vi "RX JESD Sync.vi"(0 "rx baseband session in":T2={"3630 session"={"VISA resource name"="", "Address Space"=1, "window_offset"=0, "register_addresses"={"MM based Registers"={"Revision"=0, "OldestCompatRev"=0, "signature"=0, "scratch"=0, "LedControl"=0, "BoardHwRev"=0, "BoardControl"=0, "ThermalStatus"=0, "BasebandStatus"=0, "BasebandControl"=0, "BasebandAuxSetup"=0, "BasebandAuxStatus"=0, "LmkSyncOutSetup"=0, " AdcSyncOutSetup"=0, " InjSyncOutSetup"=0, " PxiTrig0OutSetup"=0, " PxiTrig1OutSetup"=0, " PxiTrig2OutSetup"=0, " PxiTrig3OutSetup"=0, " PxiTrig4OutSetup"=0, " PxiTrig5OutSetup"=0, " PxiTrig6OutSetup"=0, " PxiTrig7OutSetup"=0}, "CPLD based Registers"={"SlaveSignature"=0, "SlaveRevision"=0, "SlaveOldestCompatRev"=0, "SlaveScratch"=0, "SlaveSetup"=0, "SlaveStatus"=0, "IDacReg_offset"=0, "LMKRegGrp0_offset"=0, "QDacReg_offset"=0, "BrdTempSensorVal"=0, "TempSensorPowerDown"=0, "GPIOReg_offset"=0, "IAdcReg_offset"=0, "QAdcReg_offset"=0, "LMKRegGrp1_offset"=0, "QadcTempSensorVal"=0, "IadcTempSensorVal"=0, "RevisionReg"=0, "VcxoReg"=0, "CpldStatusReg"=0, "PowerReg"=0, "VBiasEnReg"=0, "ExtRefOeReg"=0, "QdacCtrlReg"=0, "QdacStatusReg"=0, "IdacCtrlReg"=0, "IdacStatusReg"=0, "QdacJtagIn"=0, "QdacJtagOut"=0, "IdacJtagIn"=0, "IdacJtagOut"=0, "IqDcSetupReg"=0, "QadcStatusReg"=0, "IadcStatusReg"=0, "BrdSetupReg"=0, "IqDcRevisionReg"=0, "PllStatusReg"=0, "EndpointScratchReg"=0, "AdcSyncCfgReg"=0, "IqCardOpampReg"=0}, "CPLD Register Offset"=0, "MM  Register Offset"=0, " PxiTrig0OutSetup"=0}, "required_MM_fpga_version"={"signature"=0, "hardware"=0, "current revision"=0, "oldest revision"=0}, "CPLD Oldest Compat Version "={"hardware"=0, "CPLD firmware"=0}, "MM_FPGA_image_location"="", "is_init"=FALSE, "card_type"=enum."ADC", "DacLmkConfigFileName"="", "AdcLmkConfigFileName"="", "AdcConfigFileName"="", "DacConfigFileName_RevA"="", "DacConfigFileName_RevB"="", "Mulde hardware revision"=0, "bypass DAC PLL\n"=FALSE, "IQ Card Revision"=enum."RevA", "board capability"={"baseband sync"=enum."no baseband sync"}}, "7902 reference"=refnum} {"3630 session"."Address Space" items=["VXI/VME A16"=1, "VXI/VME A24"=2, "VXI/VME A32"=3, "VXI/VME A64"=4, "PXI Memory Allocations"=9, "PXI Configuration"=10, "PXI BAR0"=11, "PXI BAR1"=12, "PXI BAR2"=13, "PXI BAR3"=14, "PXI BAR4"=15, "PXI BAR5"=16]}, 5 "fpga reference in":refnum<k20>[](array[refnum]), 7 "direction":T1, 9 "timeout (ms)":dbl=500.0 format="%#_13g", 11 "error in":errorcluster) -> (4 "rx baseband session out":T2={"3630 session"={"VISA resource name"="", "Address Space"=1, "window_offset"=0, "register_addresses"={"MM based Registers"={"Revision"=0, "OldestCompatRev"=0, "signature"=0, "scratch"=0, "LedControl"=0, "BoardHwRev"=0, "BoardControl"=0, "ThermalStatus"=0, "BasebandStatus"=0, "BasebandControl"=0, "BasebandAuxSetup"=0, "BasebandAuxStatus"=0, "LmkSyncOutSetup"=0, " AdcSyncOutSetup"=0, " InjSyncOutSetup"=0, " PxiTrig0OutSetup"=0, " PxiTrig1OutSetup"=0, " PxiTrig2OutSetup"=0, " PxiTrig3OutSetup"=0, " PxiTrig4OutSetup"=0, " PxiTrig5OutSetup"=0, " PxiTrig6OutSetup"=0, " PxiTrig7OutSetup"=0}, "CPLD based Registers"={"SlaveSignature"=0, "SlaveRevision"=0, "SlaveOldestCompatRev"=0, "SlaveScratch"=0, "SlaveSetup"=0, "SlaveStatus"=0, "IDacReg_offset"=0, "LMKRegGrp0_offset"=0, "QDacReg_offset"=0, "BrdTempSensorVal"=0, "TempSensorPowerDown"=0, "GPIOReg_offset"=0, "IAdcReg_offset"=0, "QAdcReg_offset"=0, "LMKRegGrp1_offset"=0, "QadcTempSensorVal"=0, "IadcTempSensorVal"=0, "RevisionReg"=0, "VcxoReg"=0, "CpldStatusReg"=0, "PowerReg"=0, "VBiasEnReg"=0, "ExtRefOeReg"=0, "QdacCtrlReg"=0, "QdacStatusReg"=0, "IdacCtrlReg"=0, "IdacStatusReg"=0, "QdacJtagIn"=0, "QdacJtagOut"=0, "IdacJtagIn"=0, "IdacJtagOut"=0, "IqDcSetupReg"=0, "QadcStatusReg"=0, "IadcStatusReg"=0, "BrdSetupReg"=0, "IqDcRevisionReg"=0, "PllStatusReg"=0, "EndpointScratchReg"=0, "AdcSyncCfgReg"=0, "IqCardOpampReg"=0}, "CPLD Register Offset"=0, "MM  Register Offset"=0, " PxiTrig0OutSetup"=0}, "required_MM_fpga_version"={"signature"=0, "hardware"=0, "current revision"=0, "oldest revision"=0}, "CPLD Oldest Compat Version "={"hardware"=0, "CPLD firmware"=0}, "MM_FPGA_image_location"="", "is_init"=FALSE, "card_type"=enum."ADC", "DacLmkConfigFileName"="", "AdcLmkConfigFileName"="", "AdcConfigFileName"="", "DacConfigFileName_RevA"="", "DacConfigFileName_RevB"="", "Mulde hardware revision"=0, "bypass DAC PLL\n"=FALSE, "IQ Card Revision"=enum."RevA", "board capability"={"baseband sync"=enum."no baseband sync"}}, "7902 reference"=refnum} {"3630 session"."Address Space" items=["VXI/VME A16"=1, "VXI/VME A24"=2, "VXI/VME A32"=3, "VXI/VME A64"=4, "PXI Memory Allocations"=9, "PXI Configuration"=10, "PXI BAR0"=11, "PXI BAR1"=12, "PXI BAR2"=13, "PXI BAR3"=14, "PXI BAR4"=15, "PXI BAR5"=16]}, 8 "timeout error":bool, 15 "error out":errorcluster)   [LabVIEW 2019]
uses:
  TypeDefs/Rx Baseband Session.ctl
  <instrlib>/niMmWave/ni3610 and ni3630/controls/public/Main Settings.ctl
  <vilib>/Instr/_visa.llb/VISA Register Access Address Space.ctl
  <instrlib>/niMmWave/ni3610 and ni3630/controls/public/Register Adresses.ctl
  <instrlib>/niMmWave/ni3610 and ni3630/controls/public/Base Card Type.ctl
  <instrlib>/niMmWave/ni3610 and ni3630/controls/private/IQ Card Revision.ctl
  <instrlib>/niMmWave/ni3610 and ni3630/controls/public/Board Capability.ctl
  TypeDefs/Blank FPGA Reference.ctl
  TypeDefs/Direction.ctl
  TypeDefs/RX FPGA Reference.ctl
  <vilib>/rvi/errors/niLvFpgaAdjustHostInterfaceError.vi
  <vilib>/rvi/interface/nirviReadWriteControl/nirviReadWriteControl.xnode
  <vilib>/rvi/interface/Simulation/niFpgaSimulationCallBeginRW.vi
  <instrlib>/niMmWave/ni3610 and ni3630/ni3610_and_ni3630_Driver_Lib.lvlib
  NiFpgaLv.dll
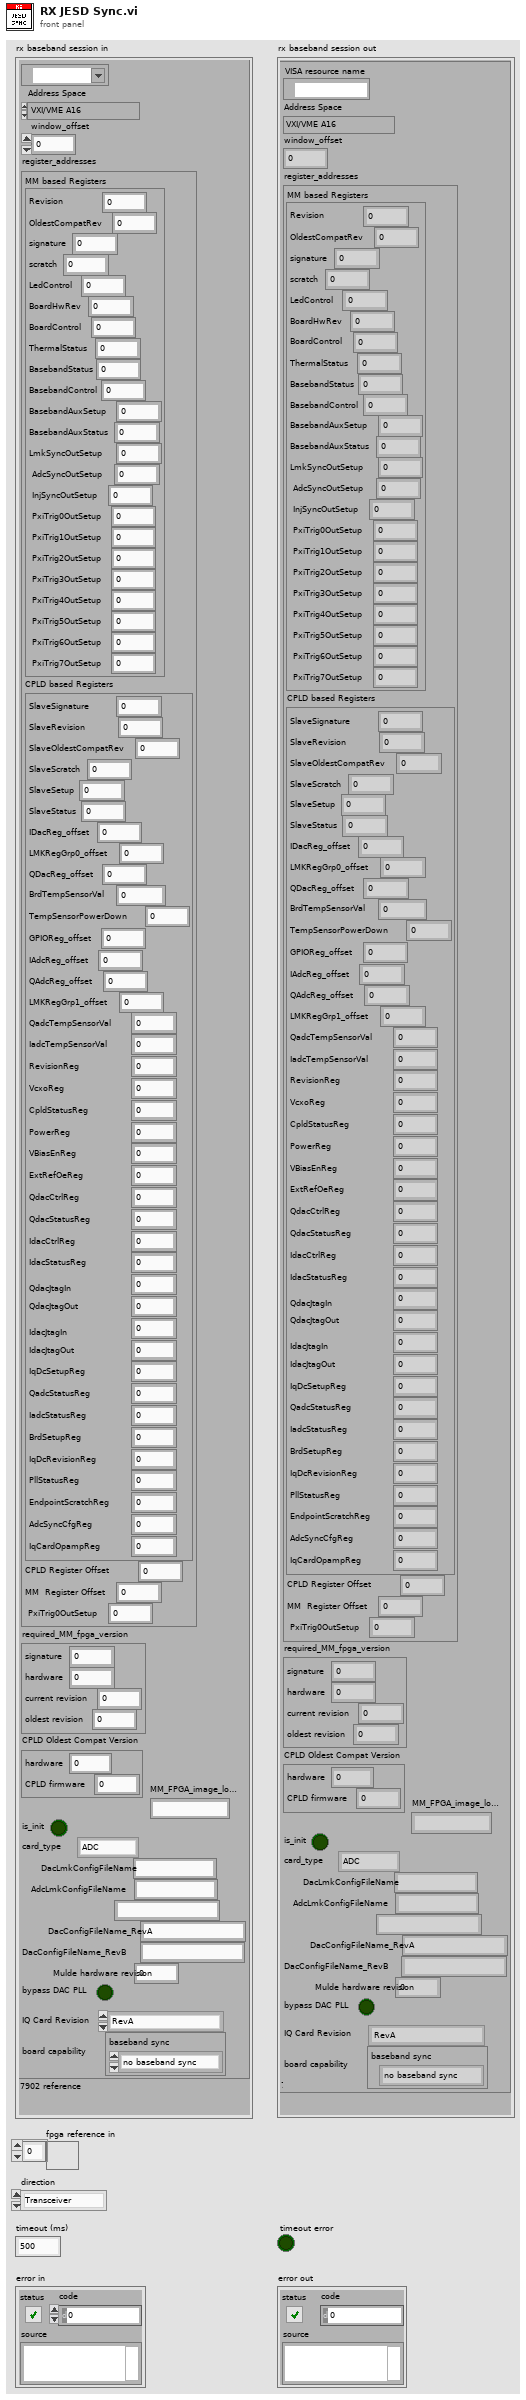
[diagram p1: front panel]
types:
  T1 = typedef "Direction.ctl" = enum16{"Transceiver", "Receiver", "Transmitter"}
  T2 = typedef "Rx Baseband Session.ctl" = cluster{"3630 session":T3, "7902 reference":T9}
  T3 = typedef "ni3610_and_ni3630_Driver_Lib.lvlib/Main Settings.ctl" = cluster{"VISA resource name":refnum<visa-resource-name>, "Address Space":T4, "window_offset":u32, "register_addresses":T5, "required_MM_fpga_version":cluster{"signature":u32, "hardware":u32, "current revision":u32, "oldest revision":u32}, "CPLD Oldest Compat Version ":cluster{"hardware":u32, "CPLD firmware":u32}, "MM_FPGA_image_location":string, "is_init":bool, "card_type":T6, "DacLmkConfigFileName":string, "AdcLmkConfigFileName":string, "AdcConfigFileName":string, "DacConfigFileName_RevA":string, "DacConfigFileName_RevB":string, "Mulde hardware revision":u8, "bypass DAC PLL\n":bool, "IQ Card Revision":T7, "board capability":T8}
  T4 = typedef "VISA Register Access Address Space.ctl" = u16
  T5 = typedef "ni3610_and_ni3630_Driver_Lib.lvlib/Register Adresses.ctl" = cluster{"MM based Registers":cluster{"Revision":u32, "OldestCompatRev":u32, "signature":u32, "scratch":u32, "LedControl":u32, "BoardHwRev":u32, "BoardControl":u32, "ThermalStatus":u32, "BasebandStatus":u32, "BasebandControl":u32, "BasebandAuxSetup":u32, "BasebandAuxStatus":u32, "LmkSyncOutSetup":u32, " AdcSyncOutSetup":u32, " InjSyncOutSetup":u32, " PxiTrig0OutSetup":u32, " PxiTrig1OutSetup":u32, " PxiTrig2OutSetup":u32, " PxiTrig3OutSetup":u32, " PxiTrig4OutSetup":u32, " PxiTrig5OutSetup":u32, " PxiTrig6OutSetup":u32, " PxiTrig7OutSetup":u32}, "CPLD based Registers":cluster{"SlaveSignature":u32, "SlaveRevision":u32, "SlaveOldestCompatRev":u32, "SlaveScratch":u32, "SlaveSetup":u32, "SlaveStatus":u32, "IDacReg_offset":u32, "LMKRegGrp0_offset":u32, "QDacReg_offset":u32, "BrdTempSensorVal":u32, "TempSensorPowerDown":u32, "GPIOReg_offset":u32, "IAdcReg_offset":u32, "QAdcReg_offset":u32, "LMKRegGrp1_offset":u32, "QadcTempSensorVal":u32, "IadcTempSensorVal":u32, "RevisionReg":u32, "VcxoReg":u32, "CpldStatusReg":u32, "PowerReg":u32, "VBiasEnReg":u32, "ExtRefOeReg":u32, "QdacCtrlReg":u32, "QdacStatusReg":u32, "IdacCtrlReg":u32, "IdacStatusReg":u32, "QdacJtagIn":u32, "QdacJtagOut":u32, "IdacJtagIn":u32, "IdacJtagOut":u32, "IqDcSetupReg":u32, "QadcStatusReg":u32, "IadcStatusReg":u32, "BrdSetupReg":u32, "IqDcRevisionReg":u32, "PllStatusReg":u32, "EndpointScratchReg":u32, "AdcSyncCfgReg":u32, "IqCardOpampReg":u32}, "CPLD Register Offset":u32, "MM  Register Offset":u32, " PxiTrig0OutSetup":u32}
  T6 = typedef "ni3610_and_ni3630_Driver_Lib.lvlib/Base Card Type.ctl" = enum16{"unspecified", "ADC", "DAC"}
  T7 = typedef "ni3610_and_ni3630_Driver_Lib.lvlib/IQ Card Revision.ctl" = enum16{"RevA", "RevB", "RevC", "RevD"}
  T8 = typedef "ni3610_and_ni3630_Driver_Lib.lvlib/Board Capability.ctl" = cluster{"baseband sync":enum16{"no baseband sync", "baseband sync"}}
  T9 = typedef "Blank FPGA Reference.ctl" = refnum<k20>
  T10 = typedef "RX FPGA Reference.ctl" = refnum<k20>
  T11 = cluster{"gtx enable":bool, "jesd enable":bool, "sw sync":bool, "buffer enable":bool, "clock enable":bool, "trig5 output enable":bool, "trig5 invert":bool}
  T12 = cluster{"gtx active":bool, "jesd active":bool, "lane sync req":bool, "lanes synced":bool, "lanes aligned":bool, "qpll locked":bool, "qpll ref lost":bool, "k-char error":bool, "lane alignment error":bool, "8b10b error":bool, "8b10b disparity error":bool, "buffer overflow":bool, "buffer underflow":bool, "buffer ready":bool, "mgt ref clocks locked":bool, "mgt ref clock valid":bool, "config complete":bool}
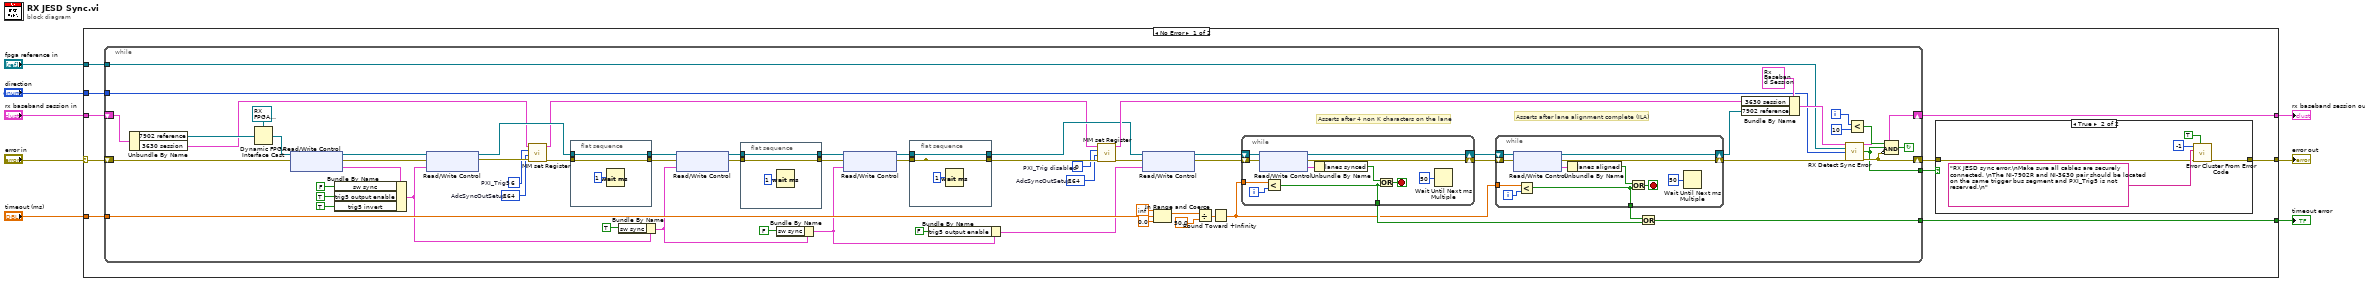
[diagram p0: block diagram]
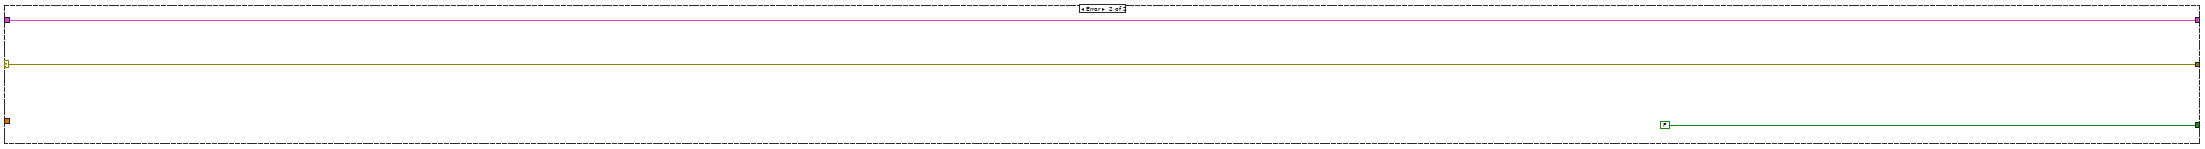
[diagram p3: hidden frame]
diagram:
  n1 = case shown="No Error" "error in" {
    selector: "error in" -> [w15 w124]
    tunnel: [w12 w124] -> w8
    tunnel: [w18 FALSE] -> w6
    tunnel: "timeout (ms)" -> [w17 _]
    tunnel: "rx baseband session in" -> [w16 w122]
    tunnel: [w11 w122] -> w3
    tunnel: "fpga reference in" -> [w10 _]
    tunnel: "direction" -> [w9 _]
    frame No Error {
      n2 = while {
        tunnel: [w80] -> w18
        tunnel: w17 -> [w79]
        shift-right: [w66] -> w13
        shift-left: w15 -> [w22]
        shift-right: [w56] -> w11
        shift-left: w16 -> [w58]
        tunnel: [w64] -> w14
        tunnel: w10 -> [w20]
        tunnel: w9 -> [w19]
        i -> [w65]
        stop <- w67 continue-if-true
        w38 = u32 0  # PXI_Trig disabled
        w37 = u32 264  # AdcSyncOutSetup
        w43 = u32 6  # PXI_Trig5
        w42 = u32 264  # AdcSyncOutSetup
        # "Asserts after lane alignment complete (ILA)"
        # "Asserts after 4 non K characters on the lane"
        n3 = Unbundle By Name(w58) -> ("7902 reference"=w60:T9, "3630 session"=w21:T3)
        n4 = Dynamic FPGA Interface Cast(Session In=T10 refnum ("fpga reference"), Type=w60) -> (Session Out=w36:T10)
        n5 = xnode "Read/Write Control"("FPGA VI Reference In"=w36, "error in"=w22) -> ("FPGA VI Reference Out"=w35:T10, "error out"=w34:errorcluster, "rxjesd.control"=w33:T11)
        n6 = Bundle By Name(cluster=w33, "sw sync"=FALSE ("txjesd.reset"), "trig5 output enable"=TRUE ("pxi trig 5 output enable"), "trig5 invert"=TRUE ("invert jesd sync to pin")) -> (w29:T11)
        n7 = xnode "Read/Write Control"("FPGA VI Reference In"=w35, "error in"=w34, "rxjesd.control"=w29) -> ("FPGA VI Reference Out"=w55:T10, "error out"=w44:errorcluster)
        n8 = call <instrlib>:"MM set Register.vi"("error in"=w44, "MM address"=w42, "Value"=w43, "Board Settings in"=w21) -> ("error out"=w45:errorcluster, "Board Settings out"=w39:T3)  [unwired: 6 in]
        n9 = flat-sequence {
          tunnel: w55 -> [w89]
          tunnel: w45 -> [w88]
          tunnel: [w89] -> w48
          tunnel: [w88] -> w49
          frame #0 {
            n10 = Wait (ms)(milliseconds to wait=u32 1) -> ()  [unwired: 1 out]
          }
        }
        n11 = Bundle By Name(cluster=w29, "sw sync"=TRUE ("rxjesd.sw sync")) -> (w25:T11)
        n12 = xnode "Read/Write Control"("FPGA VI Reference In"=w48, "error in"=w49, "rxjesd.control"=w25) -> ("FPGA VI Reference Out"=w52:T10, "error out"=w53:errorcluster)
        n13 = flat-sequence {
          tunnel: w52 -> [w92]
          tunnel: w53 -> [w91]
          tunnel: [w92] -> w51
          tunnel: [w91] -> w50
          frame #0 {
            n14 = Wait (ms)(milliseconds to wait=u32 1) -> ()  [unwired: 1 out]
          }
        }
        n15 = Bundle By Name(cluster=w25, "sw sync"=FALSE ("rxjesd.sw sync")) -> (w23:T11)
        n16 = xnode "Read/Write Control"("FPGA VI Reference In"=w51, "error in"=w50, "rxjesd.control"=w23) -> ("FPGA VI Reference Out"=w46:T10, "error out"=w47:errorcluster)
        n17 = flat-sequence {
          tunnel: w46 -> [w86]
          tunnel: [w85] -> _
          tunnel: [w86] -> w54
          tunnel: [w85] -> w40
          tunnel: w47 -> [w85]
          frame #0 {
            n18 = Wait (ms)(milliseconds to wait=u32 1) -> ()  [unwired: 1 out]
          }
        }
        n19 = Bundle By Name(cluster=w23, "trig5 output enable"=FALSE ("rxjesd.sw sync")) -> (w24:T11)
        n20 = call <instrlib>:"MM set Register.vi"("error in"=w40, "MM address"=w37, "Value"=w38, "Board Settings in"=w39) -> ("error out"=w41:errorcluster, "Board Settings out"=w63:T3)  [unwired: 6 in]
        n21 = xnode "Read/Write Control"("FPGA VI Reference In"=w54, "error in"=w41, "rxjesd.control"=w24) -> ("FPGA VI Reference Out"=w72:T10, "error out"=w71:errorcluster)
        n22 = In Range and Coerce(upper limit=inf, x=w79, lower limit=0.0) -> (coerced(x)=w76:dbl)  [unwired: 1 out]
        n23 = Divide(x=w76, y=50.0) -> (x/y=w74:dbl)
        n24 = Round Toward +Infinity(x=w74) -> (ceil(x): smallest int >= x=w73:dbl)
        n25 = while {
          shift-right: [w100] -> w83
          shift-left: w71 -> [w102]
          shift-right: [w103] -> w84
          shift-left: w72 -> [w104]
          tunnel: w73 -> [w97]
          tunnel: [w96] -> w82
          i -> [w99]
          stop <- w98 stop-if-true
          n26 = xnode "Read/Write Control"("FPGA VI Reference In"=w104, "error in"=w102) -> ("FPGA VI Reference Out"=w103:T10, "error out"=w100:errorcluster, "rxjesd.status"=w95:T12)
          n27 = Less?(x=w97, y=w99) -> (x < y?=w96:bool)
          n28 = Unbundle By Name(w95) -> ("lanes synced"=w94:bool)
          n29 = Or(x=w94, y=w96) -> (x .or. y?=w98:bool)
          n30 = Wait Until Next ms Multiple(millisecond multiple=u32 50) -> ()  [unwired: 1 out]
        }
        n31 = while {
          shift-right: [w112] -> w70
          shift-left: w83 -> [w113]
          shift-right: [w114] -> w61
          shift-left: w84 -> [w115]
          tunnel: w73 -> [w109]
          tunnel: [w108] -> w81
          i -> [w111]
          stop <- w110 stop-if-true
          n32 = xnode "Read/Write Control"("FPGA VI Reference In"=w115, "error in"=w113) -> ("FPGA VI Reference Out"=w114:T10, "error out"=w112:errorcluster, "rxjesd.status"=w106:T12)
          n33 = Less?(x=w109, y=w111) -> (x < y?=w108:bool)
          n34 = Unbundle By Name(w106) -> ("lanes aligned"=w105:bool)
          n35 = Or(x=w105, y=w108) -> (x .or. y?=w110:bool)
          n36 = Wait Until Next ms Multiple(millisecond multiple=u32 50) -> ()  [unwired: 1 out]
        }
        n37 = Or(x=w81, y=w82) -> (x .or. y?=w80:bool)
        n38 = Bundle By Name(cluster=T2 {"3630 session"={"VISA resource name"="", "Address Space"=1, "window_offset"=0, "register_addresses"={"MM based Registers"={"Revision"=0, "OldestCompatRev"=0, "signature"=0, "scratch"=0, "LedControl"=0, "BoardHwRev"=0, "BoardControl"=0, "ThermalStatus"=0, "BasebandStatus"=0, "BasebandControl"=0, "BasebandAuxSetup"=0, "BasebandAuxStatus"=0, "LmkSyncOutSetup"=0, " AdcSyncOutSetup"=0, " InjSyncOutSetup"=0, " PxiTrig0OutSetup"=0, " PxiTrig1OutSetup"=0, " PxiTrig2OutSetup"=0, " PxiTrig3OutSetup"=0, " PxiTrig4OutSetup"=0, " PxiTrig5OutSetup"=0, " PxiTrig6OutSetup"=0, " PxiTrig7OutSetup"=0}, "CPLD based Registers"={"SlaveSignature"=0, "SlaveRevision"=0, "SlaveOldestCompatRev"=0, "SlaveScratch"=0, "SlaveSetup"=0, "SlaveStatus"=0, "IDacReg_offset"=0, "LMKRegGrp0_offset"=0, "QDacReg_offset"=0, "BrdTempSensorVal"=0, "TempSensorPowerDown"=0, "GPIOReg_offset"=0, "IAdcReg_offset"=0, "QAdcReg_offset"=0, "LMKRegGrp1_offset"=0, "QadcTempSensorVal"=0, "IadcTempSensorVal"=0, "RevisionReg"=0, "VcxoReg"=0, "CpldStatusReg"=0, "PowerReg"=0, "VBiasEnReg"=0, "ExtRefOeReg"=0, "QdacCtrlReg"=0, "QdacStatusReg"=0, "IdacCtrlReg"=0, "IdacStatusReg"=0, "QdacJtagIn"=0, "QdacJtagOut"=0, "IdacJtagIn"=0, "IdacJtagOut"=0, "IqDcSetupReg"=0, "QadcStatusReg"=0, "IadcStatusReg"=0, "BrdSetupReg"=0, "IqDcRevisionReg"=0, "PllStatusReg"=0, "EndpointScratchReg"=0, "AdcSyncCfgReg"=0, "IqCardOpampReg"=0}, "CPLD Register Offset"=0, "MM  Register Offset"=0, " PxiTrig0OutSetup"=0}, "required_MM_fpga_version"={"signature"=0, "hardware"=0, "current revision"=0, "oldest revision"=0}, "CPLD Oldest Compat Version "={"hardware"=0, "CPLD firmware"=0}, "MM_FPGA_image_location"="", "is_init"=FALSE, "card_type"=enum."ADC", "DacLmkConfigFileName"="", "AdcLmkConfigFileName"="", "AdcConfigFileName"="", "DacConfigFileName_RevA"="", "DacConfigFileName_RevB"="", "Mulde hardware revision"=0, "bypass DAC PLL\n"=FALSE, "IQ Card Revision"=enum."RevA", "board capability"={"baseband sync"=enum."no baseband sync"}}, "7902 reference"=refnum} ("rx baseband session out 2"), "3630 session"=w63, "7902 reference"=w61) -> (w57:T2)
        n39 = call "RX Detect Sync Error.vi"("rx baseband session in"=w57, "fpga reference in"=w20, "direction"=w19, "error in"=w70) -> ("rx baseband session out"=w56:T2, "sync error"=w64:bool, "error out"=w66:errorcluster)  [unwired: 9 in]
        n40 = Less?(x=w65, y=10) -> (x < y?=w68:bool)
        n41 = Compound Arithmetic op=AND(w68, w64, invert w66) -> (w67:bool)
      }
      n42 = case shown="True" w14 {
        tunnel: w13 -> [w116 w119]
        tunnel: [w116 w118] -> w12
        frame False {
        }
        frame True {
          n43 = call <vilib>:"Error Cluster From Error Code.vi"("show call chain? (False)"=TRUE, "error in (no error)"=w119, "error message (\"\")"="RX JESD sync error.\nMake sure all cables are securely connected. \nThe NI-7902R and NI-3630 pair should be located on the same trigger bus segment and PXI_Trig5 is not reserved.\n" ("source"), "error code (0)"=-1) -> ("error out"=w118:errorcluster)  [unwired: 5 in]
        }
      }
    }
    frame Error {
    }
  }
  "error out" <- w8
  "timeout error" <- w6
  "rx baseband session out" <- w3
